vi "ke37xx Configure DB Reference.vi"(0 "VISA Resource Name":refnum<visa-resource-name>, 7 "DB Reference (1 V)":dbl=1.0, 11 "error in (no error)":errorcluster) -> (4 "VISA Resource Name Out":refnum<visa-resource-name>, 15 "error out":errorcluster)   [LabVIEW 2009, in "Keithley 3700 Series.lvlib"]
doc: "This VI configures the DB reference value for the selected function. The DB reference only applies when the measurement function is DC Votls or AC Volts. For all other measurement functions, an error will be generated if the DB reference is set."
uses:
  <instrlib>/Keithley 3706/Keithley 3700 Series.lvlib
panel:
  # "s"
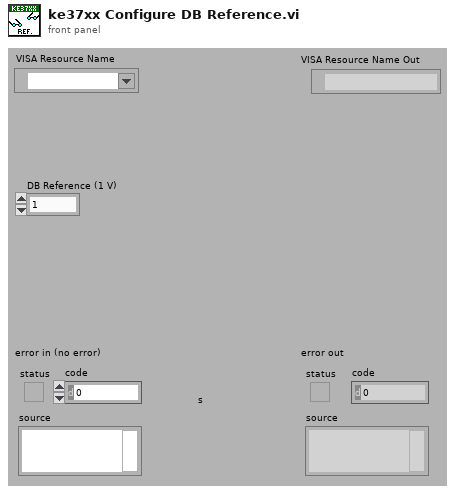
[diagram p1: front panel]
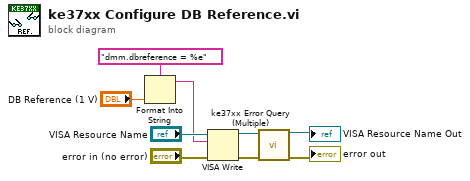
[diagram p0: block diagram]
diagram:
  n1 = Format Into String(format string="dmm.dbreference = %e" ("write buffer"), "DB Reference (1 V)") -> (resulting string=w2:string)  [unwired: 2 in, 1 out]
  n2 = VISA Write(VISA resource name="VISA Resource Name", write buffer=w2, error in (no error)="error in (no error)") -> (VISA resource name out=w5:refnum<visa-resource-name>, error out=w4:errorcluster)  [unwired: 1 out]
  n3 = call <instrlib>:"ke37xx Error Query (Multiple).vi"("VISA resource name"=w5, "error in (no error)"=w4) -> ("VISA resource name out"=→"VISA Resource Name Out":refnum<visa-resource-name>, "error out"=→"error out":errorcluster)  [unwired: 12 out]
